vi "无法预知数量的多曲线波形图表.vi"() -> ()   [LabVIEW 2012]
panel:
  in  "曲线数量":i32=3
  in  "停止":bool
  out "二维数组波形图表":dbl[][](graph)
  out "簇数据波形图表":T1(graph)
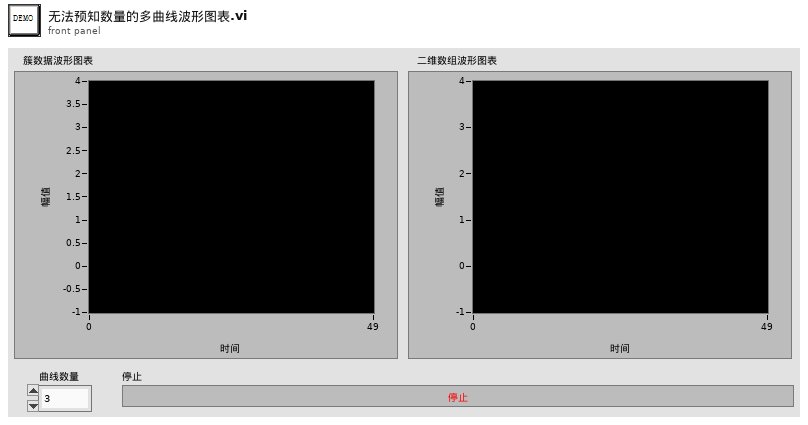
[diagram p1: front panel]
types:
  T1 = cluster{"[0]":dbl, "[1]":dbl, "[2]":dbl, "[3]":dbl, "[4]":dbl, "[5]":dbl, "[6]":dbl, "[7]":dbl, "[8]":dbl}
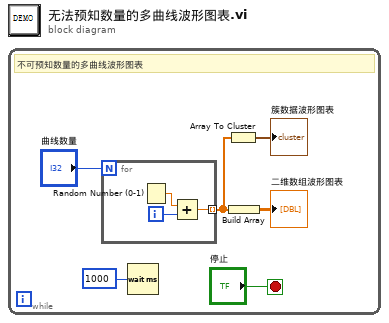
[diagram p0: block diagram]
diagram:
  n1 = while {
    stop <- "停止" stop-if-true
    # "不可预知数量的多曲线波形图表"
    n2 = for {
      N: "曲线数量" -> [_]
      tunnel: [w7] -> w1 mode=indexing
      i -> [w9]
      n3 = Random Number (0-1)() -> (number: 0 to 1=w8:dbl)
      n4 = Add(x=w8, y=w9) -> (x+y=w7:dbl)
    }
    n5 = Wait (ms)(milliseconds to wait=u32 1000 ("等待时间（毫秒）")) -> ()  [unwired: 1 out]
    n6 = Array To Cluster(array=w1) -> (cluster=→"簇数据波形图表":T1)
    n7 = Build Array(w1) -> (→"二维数组波形图表":dbl[][])
  }
